vi "Initialize.vi"(8 "error in (no error)":errorcluster, 11 "Serial in":refnum<class "Modbus Serial.lvclass">) -> (0 "error out":errorcluster, 3 "Serial out":refnum<class "Modbus Serial.lvclass">)   [LabVIEW 2021, in "Modbus Serial.lvclass"]
uses:
  Modbus Serial.lvclass
  D:/my_projects/projects/21/Master CR/Master CR.lvclass
  Param/TCP Param/TCP Param.lvclass
  Modbus_v121c/Network Protocol/Network Master/Serial/Serial Master.lvclass
  D:/my_projects/projects/21/Modbus_v121c/Network Protocol/Network Master/Network Master.lvclass
  D:/my_projects/projects/21/Modbus_v121c/Network Protocol/Network Protocol.lvclass
  Modbus_v121c/Master Function Definition/Master Function Definition.lvclass
  Modbus_v121c/Transmission Data Unit/RTU/RTU Data Unit.lvclass
  D:/my_projects/projects/21/Modbus_v121c/Transmission Data Unit/Serial Interface/Serial Data Unit.lvclass
  Modbus_v121c/Transmission Data Unit/Transmission Data Unit.lvclass/Transmission Data Unit.ctl
  Master CR.lvclass/Master CR.ctl
  Param/TCP Param/TCP Param.lvclass/TCP Param.ctl
  Modbus_v121c/Transmission Data Unit/Serial Interface/Serial Data Unit.lvclass/Serial Data Unit.ctl
  Modbus_v121c/Network Protocol/Network Master/Network Master.lvclass/Network Master.ctl
  Modbus_v121c/Transmission Data Unit/Serial Interface/Write timeout.vi
  Modbus_v121c/Transmission Data Unit/Serial Interface/Write baud rate.vi
  Modbus_v121c/Transmission Data Unit/Serial Interface/Write flow control.vi
  Modbus_v121c/Transmission Data Unit/Serial Interface/Write parity.vi
  Modbus_v121c/Transmission Data Unit/Serial Interface/Write visa resource name.vi
  Modbus_v121c/Transmission Data Unit/Serial Interface/Serial Data Unit.lvclass
  D:/my_projects/projects/21/Modbus_v121c/Transmission Data Unit/Transmission Data Unit.lvclass
  Modbus_v121c/Transmission Data Unit/ASCII/ASCII Data Unit.lvclass
  Serial.lvclass
  Modbus Serial.lvclass/Modbus Serial.ctl
  Master CR.lvclass
  Modbus_v121c/Transmission Data Unit/Transmission Data Unit.lvclass
  Modbus_v121c/Network Protocol/Network Master/Network Master.lvclass
panel:
  in  "visa resource name":refnum<visa-resource-name>
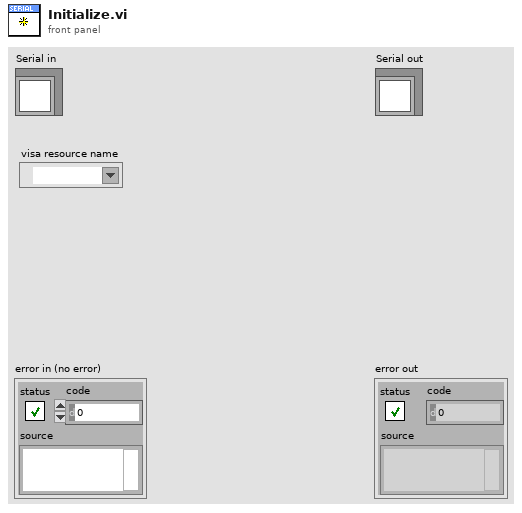
[diagram p1: front panel]
types:
  T1 = typedef "Param.lvlib/TCP Param.lvclass/timeouts.ctl" = cluster{"conn_timeout":i32, "reconn_timeout":i32, "N attempt max":i32, "t_reset_TTL":i32, "write_timeout":i32, "read_timeout":i32, "period":i32}
  T2 = cluster{"Remote IP Address":string, "Remote Port":u16}
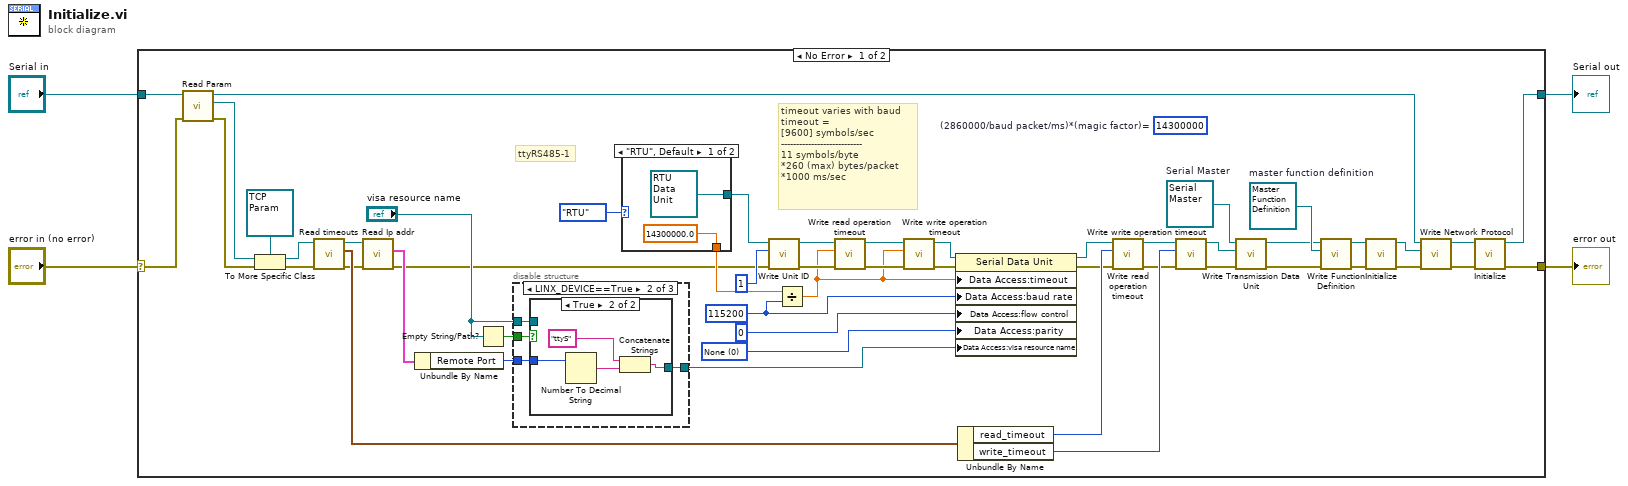
[diagram p0: block diagram]
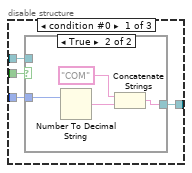
[diagram p2: hidden frame]
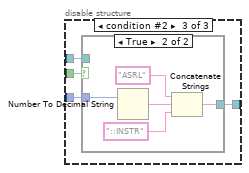
[diagram p5: hidden frame]
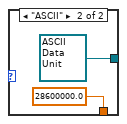
[diagram p7: hidden frame]
diagram:
  n1 = case shown="No Error" "error in (no error)" {
    selector: "error in (no error)" -> [w53 w88]
    tunnel: [w47 w88] -> w1
    tunnel: [w48 w89] -> w2
    tunnel: "Serial in" -> [w24 w89]
    frame No Error {
      w17 = refnum<class "Master Function Definition.lvclass"> refnum  # master function definition
      w23 = refnum<class "Serial Master.lvclass"> refnum  # Serial Master
      w33 = u16 0 items=["None", "Odd", "Even"] ("parity (Even)")
      w28 = u32 115200 ("baud rate (9600)")
      (unwired) u32 14300000  # (2860000/baud packet/ms)*(magic factor)=
      # "ttyRS485-1"
      # "timeout varies with baud\ntimeout =\n[9600] symbols/sec\n---------------------------\n11 symbols/byte\n*260 (max) bytes/packet\n*1000 ms/sec"
      n2 = call "Read Param.vi"("error in (no error)"=w53, "MB_TCP in"=w24) -> ("error out"=w52:errorcluster, "Param"=w50:refnum<class "Param.lvclass">, "MB_TCP out"=w22:refnum<class "Modbus Serial.lvclass">)  [unwired: 7 in]
      n3 = To More Specific Class(target class=refnum<class "TCP Param.lvclass"> refnum ("Param.lvlib:TCP Param.lvclass"), reference=w50, error in=w52) -> (specific class reference=w51:refnum<class "TCP Param.lvclass">, error out=w54:errorcluster)
      n4 = call "Read timeouts.vi"("error in (no error)"=w54, "MBParam in"=w51) -> ("error out"=w8:errorcluster, "timeouts"=w49:T1, "MBParam out"=w7:refnum<class "TCP Param.lvclass">)  [unwired: 7 in]
      n5 = call "Read Ip addr.vi"("error in (no error)"=w8, "MBParam in"=w7) -> ("error out"=w6:errorcluster, "IP address"=w11:T2)  [unwired: 7 in, 1 out]
      n6 = Unbundle By Name(w11) -> ("Remote Port"=w12:u16)
      n7 = Empty String/Path?(string/path="visa resource name") -> (empty?=w9:bool)
      n8 = disable-structure shown="LINX_DEVICE==True" {
        disable-tunnel: [w59 w65 w77] -> w5
        disable-tunnel: w9 -> [w58 w67 w76]
        disable-tunnel: "visa resource name" -> [w57 w66 w75]
        disable-tunnel: w12 -> [w56 w68 w74]
        frame condition #0 {
          n9 = case shown="True" w58 {
            tunnel: [w60 w62] -> w59
            tunnel: w57 -> [w60 _]
            tunnel: w56 -> [_ w61]
            frame False {
            }
            frame True {
              n10 = Number To Decimal String(number=w61) -> (decimal integer string=w64:string)  [unwired: 1 in]
              n11 = Concatenate Strings("COM", w64) -> (w62:string)
            }
          }
        }
        frame condition #1 (active) {
          n12 = case shown="True" w67 {
            tunnel: [w69 w71] -> w65
            tunnel: w66 -> [w69 _]
            tunnel: w68 -> [_ w70]
            frame False {
            }
            frame True {
              n13 = Number To Decimal String(number=w70) -> (decimal integer string=w73:string)  [unwired: 1 in]
              n14 = Concatenate Strings("ttyS", w73) -> (w71:string)
            }
          }
        }
        frame condition #2 {
          n15 = case shown="True" w76 {
            tunnel: [w78 w80] -> w77
            tunnel: w75 -> [w78 _]
            tunnel: w74 -> [_ w79]
            frame False {
            }
            frame True {
              n16 = Number To Decimal String(number=w79) -> (decimal integer string=w83:string)  [unwired: 1 in]
              n17 = Concatenate Strings("ASRL", w83, "::INSTR") -> (w80:string)
            }
          }
        }
      }
      n18 = case shown="\"RTU\", Default" enum16{"RTU", "ASCII"}."RTU" ("serial type") {
        tunnel: [refnum<class "RTU Data Unit.lvclass"> refnum ("RTU Data Unit") refnum<class "ASCII Data Unit.lvclass"> refnum ("ASCII Data Unit")] -> w42
        tunnel: [14300000.0 ("x") 28600000.0 ("x")] -> w37
        frame "RTU", Default {
        }
        frame "ASCII" {
        }
      }
      n19 = call "Write Unit ID.vi"("error in"=w6, "unit ID"=u8 1, "transmission data unit in"=w42) -> ("error out"=w38:errorcluster, "transmission data unit out"=w41:refnum<class "Serial Data Unit.lvclass">)  [unwired: 7 in]
      n20 = Divide(x=w37, y=w28) -> (x/y=w36:dbl)
      n21 = call "Write read operation timeout.vi"("error in (no error)"=w38, "read operation timeout"=w36, "transmission data unit in"=w41) -> ("error out"=w39:errorcluster, "transmission data unit out"=w40:refnum<class "Serial Data Unit.lvclass">)  [unwired: 7 in]
      n22 = call "Write write operation timeout.vi"("error in (no error)"=w39, "write operation timeout"=w36, "transmission data unit in"=w40) -> ("error out"=w29:errorcluster, "transmission data unit out"=w27:refnum<class "Serial Data Unit.lvclass">)  [unwired: 7 in]
      n23 = property class="Serial Data Unit"(reference=w27, error in=w29, "Data Access:timeout"=w36, "Data Access:baud rate"=w28, "Data Access:flow control"=u16 0 ("Flow Control"), "Data Access:parity"=w33, "Data Access:visa resource name"=w5) -> (reference out=w25:refnum<class "Serial Data Unit.lvclass">, error out=w26:errorcluster)
      n24 = Unbundle By Name(w49) -> ("read_timeout"=w46:i32, "write_timeout"=w45:i32)
      n25 = call "Write read operation timeout.vi"("error in (no error)"=w26, "read operation timeout"=w46, "transmission data unit in"=w25) -> ("error out"=w43:errorcluster, "transmission data unit out"=w44:refnum<class "Serial Data Unit.lvclass">)  [unwired: 7 in]
      n26 = call "Write write operation timeout.vi"("error in (no error)"=w43, "write operation timeout"=w45, "transmission data unit in"=w44) -> ("error out"=w30:errorcluster, "transmission data unit out"=w31:refnum<class "Serial Data Unit.lvclass">)  [unwired: 7 in]
      n27 = call "Write Transmission Data Unit.vi"("error in (no error)"=w30, "Transmission Data Unit"=w31, "Network Master in"=w23) -> ("error out"=w14:errorcluster, "Network Master out"=w13:refnum<class "Serial Master.lvclass">)  [unwired: 7 in]
      n28 = call "Write Function Definition.vi"("error in"=w14, "master function definition"=w17, "Modbus master in"=w13) -> ("error out"=w16:errorcluster, "Modbus master out"=w15:refnum<class "Serial Master.lvclass">)  [unwired: 7 in]
      n29 = call-dynamic "Initialize.vi"("error in"=w16, "Serial Master in"=w15) -> ("error out"=w19:errorcluster, "Serial Master out"=w18:refnum<class "Serial Master.lvclass">)  [unwired: 8 in]
      n30 = call "Write Network Protocol.vi"("error in (no error)"=w19, "Network Protocol"=w18, "Master CR in"=w22) -> ("error out"=w21:errorcluster, "Master CR out"=w20:refnum<class "Modbus Serial.lvclass">)  [unwired: 7 in]
      n31 = call-parent "Initialize.vi"("error in (no error)"=w21, "Serial in"=w20) -> ("error out"=w47:errorcluster, "Serial out"=w48:refnum<class "Modbus Serial.lvclass">)  [unwired: 8 in]
    }
    frame Error {
    }
  }
  "error out" <- w1
  "Serial out" <- w2
